vi "Eurotherm_Test.vi"() -> ()   [LabVIEW 2017]
uses:
  Eurotherm_Setpoint Control.ctl
  Eurotherm_New_Module.ctl
panel:
  in  "Address":T1(ring)
  in  "WRITE PID":bool
  in  "PID":cluster{"P":dbl, "I":dbl, "D":dbl}={"P"=50.0, "I"=120.0, "D"=600.0}
  in  "Write":T2 {"Rate (C/min)" min=0.0 max=99.9 step=0.1 format="%.1f"; "Setpoint (C)" min=-100.0 max=100.0 step=0.1 format="%.1f"}
  out "Eurotherm":T3
  in  "READ":bool
  in  "WRITE SP":bool
  in  "stop":bool
  out "error in (no error)":errorcluster
  in  "VISA resource name":refnum<visa-resource-name>="COM1"
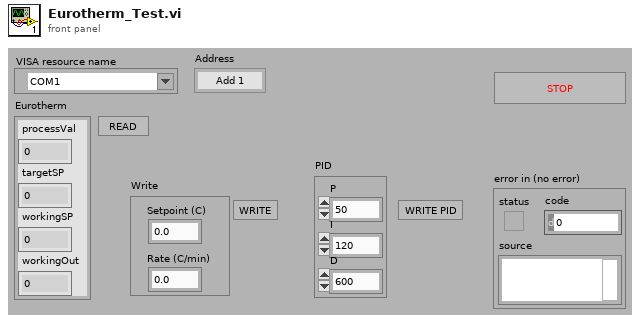
[diagram p1: front panel]
types:
  T1 = enum16{"Add 1", "Add 2", "Add 10", "Add 11", "Add 12", "Add 13"}
  T2 = typedef "Eurotherm_Setpoint Control.ctl" = cluster{"Setpoint (C)":dbl, "Rate (C/min)":dbl}
  T3 = cluster{"processVal":dbl, "targetSP":dbl, "workingSP":dbl, "workingOut":dbl}
  T4 = typedef "Eurotherm_New_Module.ctl" = enum16{"Initialize", "Write SP", "Read SP+PV", "Write Rate", "Set P", "Set I", "Set D", "Shutdown"}
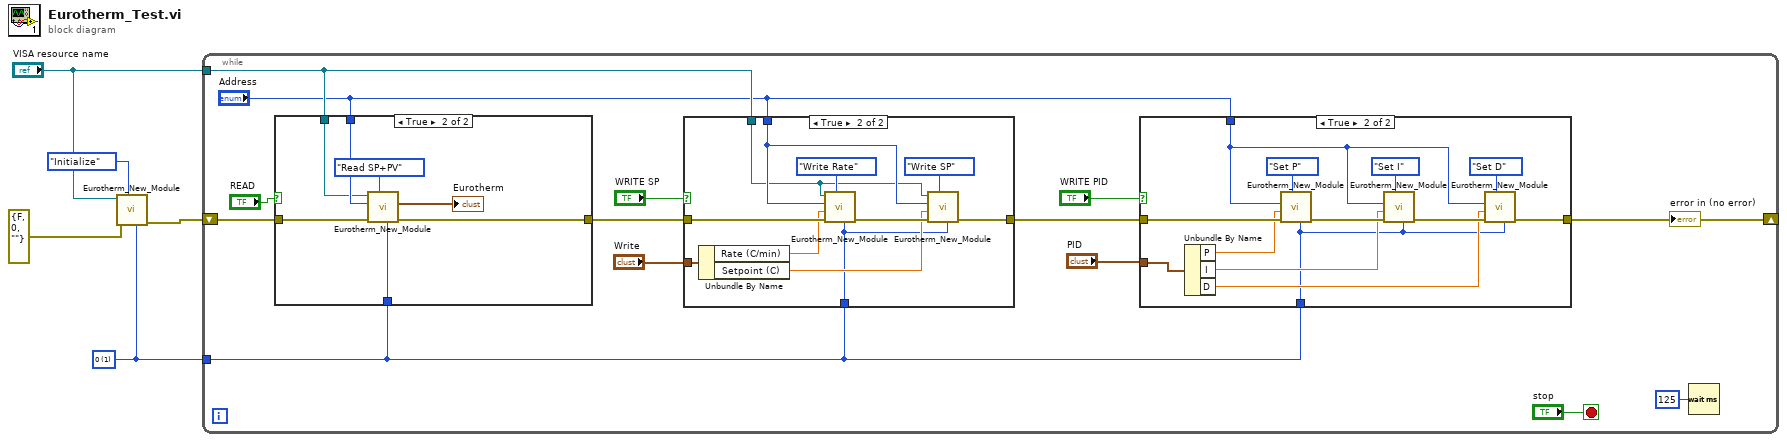
[diagram p0: block diagram]
diagram:
  w2 = u16 1 items=["0"=1, "1"=10, "2"=100] ("Decimales")
  n1 = call "Eurotherm_New_Module.vi"("Decimales"=w2, "Command"=Eurotherm_New_Module."Initialize", "error in (no error)"=errorcluster {"status"=FALSE, "code"=0, "source"=""}, "VISA resource name"="VISA resource name") -> ("error out"=w3:errorcluster)  [unwired: 6 in, 1 out]
  n2 = while {
    shift-right: [w10] -> _
    shift-left: w3 -> [w18]
    tunnel: w2 -> [w9]
    tunnel: "VISA resource name" -> [w7]
    stop <- "stop" stop-if-true
    n3 = case shown="True" "READ" {
      tunnel: w18 -> [w46 w53]
      tunnel: [w46 w52] -> w17
      tunnel: w9 -> [_ w50]
      tunnel: "Address" -> [_ w49]
      tunnel: w7 -> [_ w48]
      frame False {
      }
      frame True {
        n4 = call "Eurotherm_New_Module.vi"("Decimales"=w50, "Command"=Eurotherm_New_Module."Read SP+PV", "error in (no error)"=w53, "Address"=w49, "VISA resource name"=w48) -> ("error out"=w52:errorcluster, "Eurotherm"=→"Eurotherm":T3)  [unwired: 5 in]
      }
    }
    n5 = case shown="True" "WRITE SP" {
      tunnel: w17 -> [w34 w45]
      tunnel: [w34 w43] -> w11
      tunnel: "Write" -> [_ w40]
      tunnel: w9 -> [_ w37]
      tunnel: "Address" -> [_ w36]
      tunnel: w7 -> [_ w35]
      frame False {
      }
      frame True {
        n6 = Unbundle By Name(w40) -> ("Rate (C/min)"=w39:dbl, "Setpoint (C)"=w38:dbl)
        n7 = call "Eurotherm_New_Module.vi"("Decimales"=w37, "Command"=Eurotherm_New_Module."Write Rate", "error in (no error)"=w45, "Value"=w39, "Address"=w36, "VISA resource name"=w35) -> ("error out"=w44:errorcluster)  [unwired: 4 in, 1 out]
        n8 = call "Eurotherm_New_Module.vi"("Decimales"=w37, "Command"=Eurotherm_New_Module."Write SP", "error in (no error)"=w44, "Value"=w38, "Address"=w36, "VISA resource name"=w35) -> ("error out"=w43:errorcluster)  [unwired: 4 in, 1 out]
      }
    }
    n9 = case shown="True" "WRITE PID" {
      tunnel: w11 -> [w20 w33]
      tunnel: [w20 w24] -> w10
      tunnel: "PID" -> [_ w29]
      tunnel: w9 -> [_ w22]
      tunnel: "Address" -> [_ w21]
      frame False {
      }
      frame True {
        n10 = Unbundle By Name(w29) -> ("P"=w28:dbl, "I"=w27:dbl, "D"=w23:dbl)
        n11 = call "Eurotherm_New_Module.vi"("Decimales"=w22, "Command"=Eurotherm_New_Module."Set P", "error in (no error)"=w33, "Value"=w28, "Address"=w21) -> ("error out"=w32:errorcluster)  [unwired: 5 in, 1 out]
        n12 = call "Eurotherm_New_Module.vi"("Decimales"=w22, "Command"=Eurotherm_New_Module."Set I", "error in (no error)"=w32, "Value"=w27, "Address"=w21) -> ("error out"=w25:errorcluster)  [unwired: 5 in, 1 out]
        n13 = call "Eurotherm_New_Module.vi"("Decimales"=w22, "Command"=Eurotherm_New_Module."Set D", "error in (no error)"=w25, "Value"=w23, "Address"=w21) -> ("error out"=w24:errorcluster)  [unwired: 5 in, 1 out]
      }
    }
    "error in (no error)" <- w10
    n14 = Wait (ms)(milliseconds to wait=u32 125) -> ()  [unwired: 1 out]
  }
